vi "NiXnet DisconnectTerminals.vi"(6 "contextId":T1, 8 "error in":errorcluster, 9 "timeout (ms)":i32=-1, 10 "Request Data":T3, 11 "gRPC ID":T1) -> (0 "error out":errorcluster, 2 "Response Data":T2, 3 "gRPC ID out":T1)   [LabVIEW 2025, in "xnet-grpc_client.lvlib"]
uses:
  xnet-grpc_client.lvlib
  <vilib>/gRPC/LabVIEW gRPC Library/Shared/grpcId.ctl
  RPC Messages/nixnet_grpc_DisconnectTerminalsRequest.ctl
  RPC Messages/nixnet_grpc_DisconnectTerminalsRequest_source_enum/nixnet_grpc_DisconnectTerminalsRequest_source_enum.lvclass
  RPC Messages/nixnet_grpc_DisconnectTerminalsRequest_destination_enum/nixnet_grpc_DisconnectTerminalsRequest_destination_enum.lvclass
  RPC Messages/nidevice_grpc_Session.ctl
  RPC Messages/nixnet_grpc_DisconnectTerminalsResponse.ctl
  RPC Messages/nixnet_grpc_DisconnectTerminalsResponse_Flat.ctl
  RPC Messages/nixnet_grpc_DisconnectTerminalsRequest_source_enum/nixnet_grpc_DisconnectTerminalsRequest_source_enum.lvclass/nixnet_grpc_DisconnectTerminalsRequest_source_enum.ctl
  RPC Messages/nixnet_grpc_DisconnectTerminalsRequest_destination_enum/nixnet_grpc_DisconnectTerminalsRequest_destination_enum.lvclass/nixnet_grpc_DisconnectTerminalsRequest_destination_enum.ctl
  14035477-4c25-4107-8ed5-d0c4ef420ce5.vi
  RPC Messages/RichToFlatnidevice_grpc_Session.vi
  RPC Messages/nixnet_grpc_DisconnectTerminalsRequest_source_enum/GetActiveFieldIndex.vi
  RPC Messages/nixnet_grpc_DisconnectTerminalsRequest_source_enum/Getsource_mapped.vi
  RPC Messages/nixnet_grpc_DisconnectTerminalsRequest_source_enum/Getsource_raw.vi
  RPC Messages/nixnet_grpc_DisconnectTerminalsRequest_destination_enum/GetActiveFieldIndex.vi
  RPC Messages/nixnet_grpc_DisconnectTerminalsRequest_destination_enum/Getdestination_mapped.vi
  RPC Messages/nixnet_grpc_DisconnectTerminalsRequest_destination_enum/Getdestination_raw.vi
  <vilib>/gRPC/LabVIEW gRPC Library/Shared/TranslateGrpcError.vi
  <vilib>/gRPC/LabVIEW gRPC Library/Shared/Wait On Occurrence Wrapper.vi
  <vilib>/gRPC/LabVIEW gRPC Library/Shared/Wait On Occurence.vi
  <vilib>/gRPC/LabVIEW gRPC Library/Server API/Server/Get Server DLL Path.vi
  <vilib>/Utility/error.llb/Error Cluster From Error Code.vi
  <vilib>/Utility/config.llb/Open Config Data.vi
  <vilib>/Utility/config.llb/Write Key.vi
  <vilib>/Utility/config.llb/Write Key (Boolean).vi
  <vilib>/Utility/config.llb/Not A Config Data Refnum.vi
  <vilib>/Utility/config.llb/Read Key.vi
  <vilib>/Utility/config.llb/Read Key (Boolean).vi
  <vilib>/Utility/config.llb/Close Config Data.vi
  <vilib>/gRPC/LabVIEW gRPC Library/grpc-lvsupport-release.lvlib
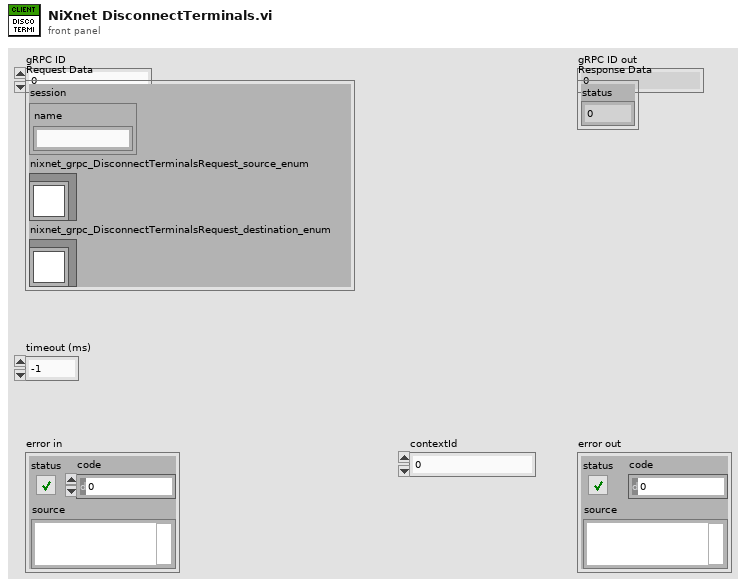
[diagram p1: front panel]
types:
  T1 = typedef "grpc-lvsupport-release.lvlib/grpcId.ctl" = u64
  T2 = typedef "xnet-grpc_client.lvlib/nixnet_grpc_DisconnectTerminalsResponse.ctl" = cluster{"status":i32}
  T3 = typedef "xnet-grpc_client.lvlib/nixnet_grpc_DisconnectTerminalsRequest.ctl" = cluster{"session":T4, "nixnet_grpc_DisconnectTerminalsRequest_source_enum":refnum<class "nixnet_grpc_DisconnectTerminalsRequest_source_enum.lvclass">, "nixnet_grpc_DisconnectTerminalsRequest_destination_enum":refnum<class "nixnet_grpc_DisconnectTerminalsRequest_destination_enum.lvclass">}
  T4 = typedef "xnet-grpc_client.lvlib/nidevice_grpc_Session.ctl" = cluster{"name":string}
  T5 = typedef "xnet-grpc_client.lvlib/nixnet_grpc_DisconnectTerminalsResponse_Flat.ctl" = cluster{"status":i32}
  T6 = typedef "xnet-grpc_client.lvlib/nixnet_grpc_DisconnectTerminalsRequest_Flat.ctl" = cluster{"session":T7, "nixnet_grpc_DisconnectTerminalsRequest_source_enum_selected_index":i32, "source_mapped":T8, "source_raw":string, "nixnet_grpc_DisconnectTerminalsRequest_destination_enum_selected_index":i32, "destination_mapped":T8, "destination_raw":string}
  T7 = typedef "xnet-grpc_client.lvlib/nidevice_grpc_Session_Flat.ctl" = cluster{"name":string}
  T8 = typedef "xnet-grpc_client.lvlib/nixnet_grpc_TerminalName.ctl" = enum32{"TERMINAL_NAME_UNSPECIFIED", "TERMINAL_NAME_PXI_TRIG_0", "TERMINAL_NAME_PXI_TRIG_1", "TERMINAL_NAME_PXI_TRIG_2", "TERMINAL_NAME_PXI_TRIG_3", "TERMINAL_NAME_PXI_TRIG_4", "TERMINAL_NAME_PXI_TRIG_5", "TERMINAL_NAME_PXI_TRIG_6", "TERMINAL_NAME_PXI_TRIG_7", "TERMINAL_NAME_FRONT_PANEL_0", "TERMINAL_NAME_FRONT_PANEL_1", "TERMINAL_NAME_PXI_STAR", "TERMINAL_NAME_PXI_CLK_10", "TERMINAL_NAME_10_MHZ_TIMEBASE", "TERMINAL_NAME_1_MHZ_TIMEBASE", "TERMINAL_NAME_MASTER_TIMEBASE", "TERMINAL_NAME_COMM_TRIGGER", "TERMINAL_NAME_START_TRIGGER", "TERMINAL_NAME_FLEX_RAY_START_CYCLE", "TERMINAL_NAME_FLEX_RAY_MACROTICK", "TERMINAL_NAME_LOG_TRIGGER", "TERMINAL_NAME_TIME_TRIGGER", "TERMINAL_NAME_NETWORK_TIME_PPS", "TERMINAL_NAME_NETWORK_TIME_1_MHZ"}
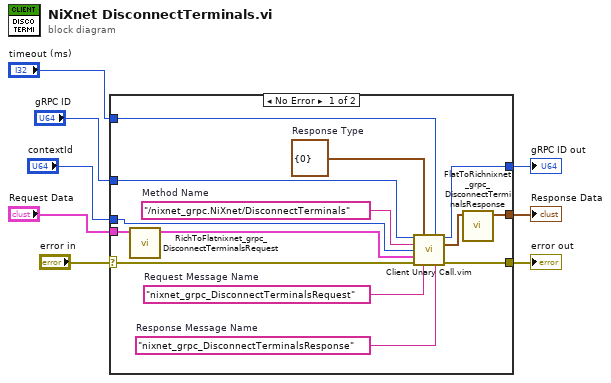
[diagram p0: block diagram]
diagram:
  n1 = case shown="No Error" "error in" {
    selector: "error in" -> [w18 w23]
    tunnel: [w17 w23] -> w7
    tunnel: "gRPC ID" -> [w16 w24]
    tunnel: [w15 w24] -> w5
    tunnel: "Request Data" -> [w12 _]
    tunnel: [w9 _] -> w3
    tunnel: "timeout (ms)" -> [w14 _]
    tunnel: "contextId" -> [w13 _]
    frame No Error {
      w19 = "nixnet_grpc_DisconnectTerminalsResponse"  # Response Message Name
      w20 = "nixnet_grpc_DisconnectTerminalsRequest"  # Request Message Name
      w21 = T5 {"status"=0}  # Response Type
      w22 = "/nixnet_grpc.NiXnet/DisconnectTerminals"  # Method Name
      n2 = call "RichToFlatnixnet_grpc_DisconnectTerminalsRequest.vi"("InputCluster"=w12) -> ("OutputCluster"=w11:T6)  [unwired: 10 in]
      n3 = call "Client Unary Call.vim"("ClientID in"=w16, "Response Type"=w21, "timeout (ms)"=w14, "Method Name"=w22, "contextId"=w13, "Request Data"=w11, "error in"=w18, "Request Message Name"=w20, "Response Message Name"=w19) -> ("ClientID out"=w15:u64, "Response Data"=w10:T5, "error out"=w17:errorcluster)  [unwired: 4 in]
      n4 = call "FlatToRichnixnet_grpc_DisconnectTerminalsResponse.vi"("InputCluster"=w10) -> ("OutputCluster"=w9:T2)  [unwired: 10 in]
    }
    frame Error {
    }
  }
  "error out" <- w7
  "gRPC ID out" <- w5
  "Response Data" <- w3
